vi "return_position.vi"(0 "from":enum16{"l", "r"}(ring), 1 "pick_drop":enum16{"pick", "drop"}(ring), 2 "is_next":bool) -> ()   [LabVIEW 2017]
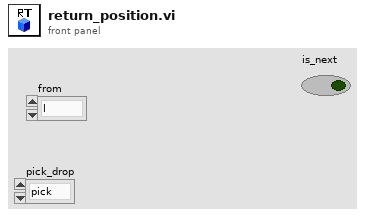
[diagram p1: front panel]
types:
  T1 = enum16{"hold", "f", "fl", "fr", "l", "r", "b", "bl", "br"}
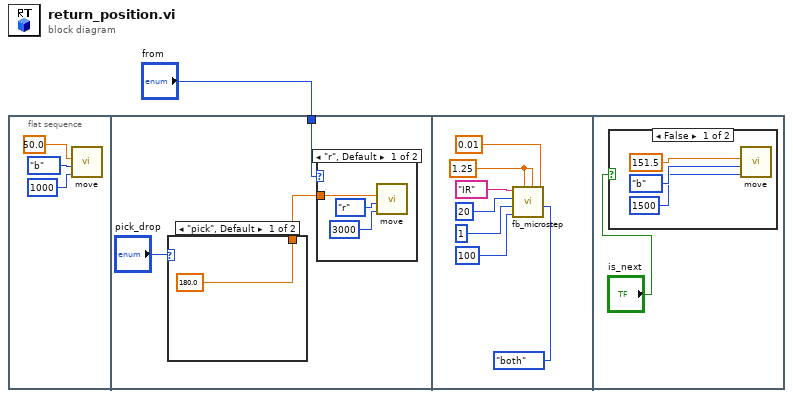
[diagram p0: block diagram]
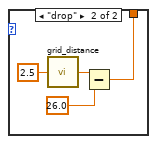
[diagram p2: hidden frame]
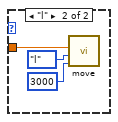
[diagram p3: hidden frame]
diagram:
  n1 = flat-sequence {
    tunnel: "from" -> [w7]
    frame #0 {
      n2 = call "move.vi"("delay"=u32 1000, "Enum"=T1."b", "D"=50.0) -> ()  [unwired: 9 in]
    }
    frame #1 {
      n3 = case shown="\"pick\", Default" "pick_drop" {
        tunnel: [180.0 ("D") w10] -> w5
        frame "pick", Default {
        }
        frame "drop" {
          n4 = call "grid_distance.vi"("x"=2.5) -> ("distance_mm"=w12:dbl)
          n5 = Subtract(x=w12, y=26.0) -> (x-y=w10:dbl)
        }
      }
      n6 = case shown="\"r\", Default" w7 {
        tunnel: w5 -> [w13 w16]
        frame "r", Default {
          n7 = call "move.vi"("delay"=u32 3000, "Enum"=T1."r", "D"=w13) -> ()  [unwired: 9 in]
        }
        frame "l" {
          n8 = call "move.vi"("delay"=u32 3000, "Enum"=T1."l", "D"=w16) -> ()  [unwired: 9 in]
        }
      }
    }
    frame #2 {
      w25 = 1.25 ("taget_IR_R")
      n9 = call "fb_microstep.vi"("Sensor"=enum16{"l", "r", "both"}."both", "precision"=0.01, "taget_IR_L"=w25, "taget_IR_R"=w25, "SamplingNUM"=100, "Step"=1, "Delay"=20, "Stop Mode"="IR") -> ()  [unwired: 3 in, 1 out]
    }
    frame #3 {
      n10 = case shown="False" "is_next" {
        frame False {
          n11 = call "move.vi"("delay"=u32 1500, "Enum"=T1."b", "D"=151.5) -> ()  [unwired: 9 in]
        }
        frame True {
        }
      }
    }
  }
